vi "MainTagBrowser.vi"() -> ()   [LabVIEW 2020]
doc: "Read Binary File opens and reads an existing file stored as a double precision array in binary form. This VI shows the simplest way to read this entire file, with the simplest error checking."
panel:
  in  "Tag List":i32(listbox)=-1
  out "TagValue":string
  out "TagName":string
  out "TagType":string
  in  "Tag_num":i32 min=0 max=106
  out "n_hdr_items":i32=80
  out "file error status":errorcluster
  out "Version":string
  out "Magic":string
  # "Select the tag number here and see the content below"
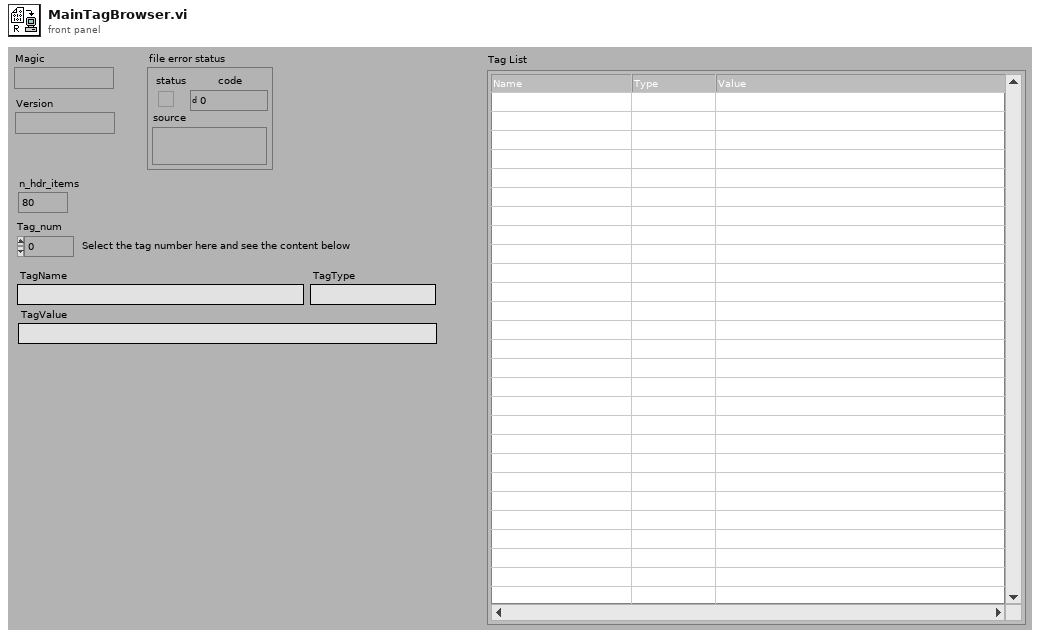
[diagram p1: front panel]
types:
  T1 = cluster{"TagIdent":string, "TagIndex":i32, "TagType":i32, "TagValue":i64, "TagAuxData":string}
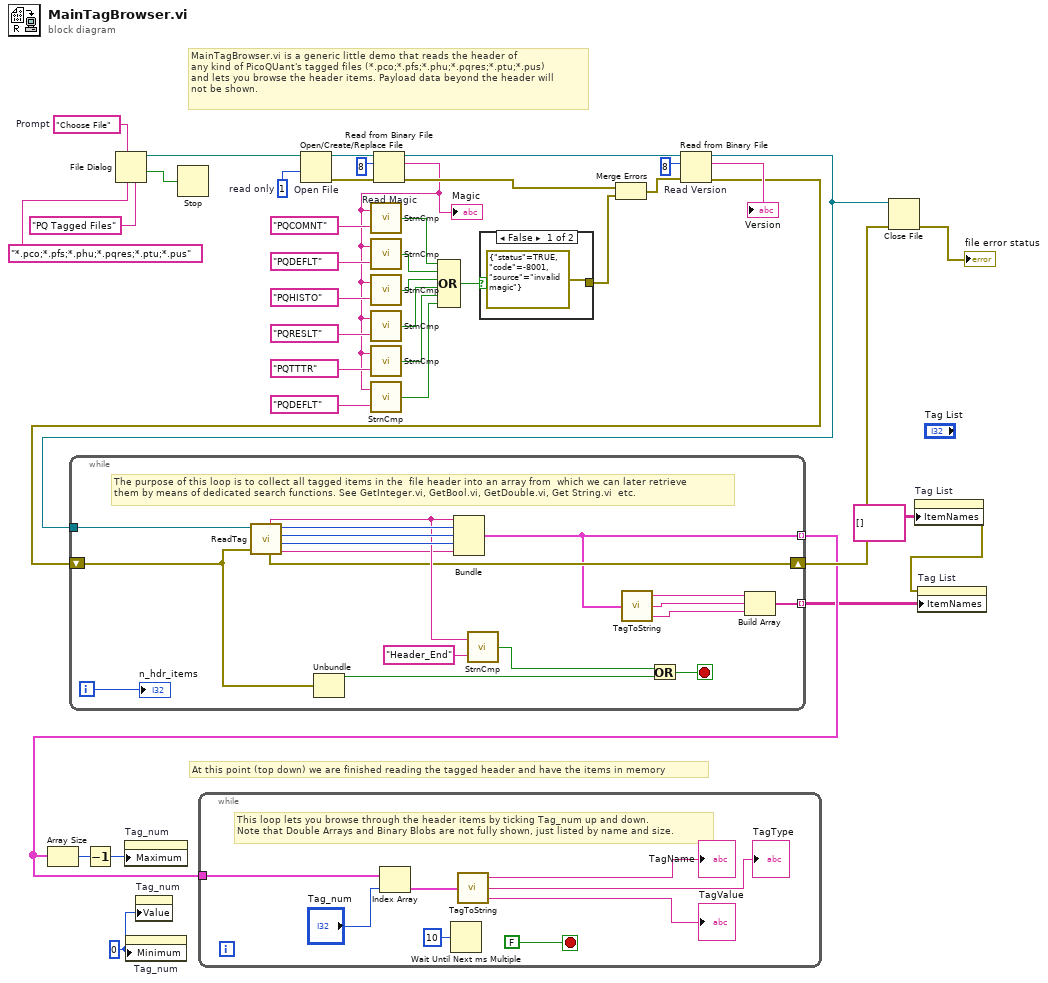
[diagram p0: block diagram]
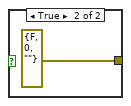
[diagram p2: hidden frame]
diagram:
  w5 = 0
  w4 = 1  # read only
  w39 = "Choose File"  # Prompt
  # "MainTagBrowser.vi is a generic little demo that reads the header of\nany kind of PicoQUant's tagged files (*.pco;*.pfs;*.phu;*.pqres;*.ptu;*.pus)\nand lets you browse the header items. Payload data beyond the header will \nnot be shown."
  # "At this point (top down) we are finished reading the tagged header and have the items in memory"
  n1 = File Dialog(4:"PQ Tagged Files", 6:"*.pco;*.pfs;*.phu;*.pqres;*.ptu;*.pus", 7:w39) -> (1:w27:bool, 3:w40:path)  [unwired: 4 in, 2 out]
  n2 = property on="Tag_num" class="DigNum (strict)"("Minimum"=w5) -> ()  [unwired: 2 in, 2 out]
  n3 = property on="Tag_num" class="DigNum (strict)"("Value"=w5) -> ()  [unwired: 2 in, 2 out]
  n4 = Stop(stop? (T)=w27) -> ()
  n5 = Open/Create/Replace File "Open File"(file path (use dialog)=w40, access (0:read/write)=w4) -> (refnum out=w29:refnum<file>, error out=w28:errorcluster)  [unwired: 4 in, 1 out]
  n6 = Read from Binary File "Read Magic"(8:w28, 10:8, 11:w29) -> (0:w33:errorcluster, 2:w9:string, 3:w38:refnum<file>)  [unwired: 3 in, 1 out]
  "Magic" <- w9
  n7 = call "StrnCmp.vi"("String 2"="PQCOMNT", "String 1"=w9) -> ("equal"=w16:bool)
  n8 = call "StrnCmp.vi"("String 2"="PQDEFLT", "String 1"=w9) -> ("equal"=w15:bool)
  n9 = call "StrnCmp.vi"("String 2"="PQHISTO", "String 1"=w9) -> ("equal"=w14:bool)
  n10 = call "StrnCmp.vi"("String 2"="PQRESLT", "String 1"=w9) -> ("equal"=w13:bool)
  n11 = call "StrnCmp.vi"("String 2"="PQTTTR", "String 1"=w9) -> ("equal"=w12:bool)
  n12 = call "StrnCmp.vi"("String 2"="PQDEFLT", "String 1"=w9) -> ("equal"=w11:bool)
  n13 = Compound Arithmetic op=OR(w16, w15, w14, w13, w12, w11) -> (w10:bool)
  n14 = case shown="False" w10 {
    tunnel: [errorcluster {"status"=TRUE, "code"=-8001, "source"="invalid magic"} ("file error status 2") errorcluster {"status"=FALSE, "code"=0, "source"=""} ("file error status 2")] -> w31
    frame False {
    }
    frame True {
    }
  }
  n15 = Merge Errors(w33, w31) -> (w32:errorcluster)
  n16 = Read from Binary File "Read Version"(8:w32, 10:8, 11:w38) -> (0:w26:errorcluster, 2:→"Version":string, 3:w24:refnum<file>)  [unwired: 3 in, 1 out]
  n17 = while {
    shift-left: w26 -> [w58]
    shift-right: [w48] -> w25
    tunnel: w24 -> [w60]
    tunnel: [w47] -> w8 mode=indexing
    tunnel: [w43] -> w3 mode=indexing
    i -> [w54]
    stop <- w59 stop-if-true
    # "The purpose of this loop is to collect all tagged items in the  file header into an array from  which we can later retrieve \nthem by means of dedicated search functions. See GetInteger.vi, GetBool.vi, GetDouble.vi, Get String.vi  etc."
    n18 = call "ReadTag.vi"("refnum"=w60, "error in"=w58) -> ("TagIdent"=w50:string, "TagIndex"=w57:i32, "TagType"=w56:i32, "error out"=w48:errorcluster, "TagValue"=w55:i64, "TagAuxData"=w49:string)  [unwired: 3 in]
    n19 = Unbundle(w58) -> ("status"=w51:bool)  [unwired: 2 out]
    n20 = Bundle("TagIdent"=w50, "TagIndex"=w57, "TagType"=w56, "TagValue"=w55, "TagAuxData"=w49) -> (w47:T1)  [unwired: 1 in]
    n21 = call "StrnCmp.vi"("String 2"="Header_End", "String 1"=w50) -> ("equal"=w52:bool)
    n22 = call "TagToString.vi"("TagData"=w47) -> ("StrTagValue"=w44:string, "StrTagType"=w45:string, "StrTagName"=w46:string)  [unwired: 2 in]
    n23 = Or(x=w52, y=w51) -> (x .or. y?=w59:bool)
    n24 = Build Array(w46, w45, w44) -> (w43:string[])
    "n_hdr_items" <- w54
  }
  n25 = Array Size(array=w8) -> (size(s)=w7:i32)
  n26 = Decrement(x=w7) -> (x-1=w6:i32)
  n27 = property on="Tag_num" class="DigNum (strict)"("Maximum"=w6) -> ()  [unwired: 2 in, 2 out]
  n28 = while {
    tunnel: w8 -> [w67]
    stop <- FALSE stop-if-true
    # "This loop lets you browse through the header items by ticking Tag_num up and down.\nNote that Double Arrays and Binary Blobs are not fully shown, just listed by name and size."
    n29 = Index Array(array=w67, index="Tag_num") -> (element=w65:T1)
    n30 = Wait Until Next ms Multiple(millisecond multiple=u32 10) -> ()  [unwired: 1 out]
    n31 = call "TagToString.vi"("TagData"=w65) -> ("StrTagValue"=→"TagValue":string, "StrTagType"=→"TagType":string, "StrTagName"=→"TagName":string)  [unwired: 2 in]
  }
  n32 = Close File(refnum=w24, error in=w25) -> (error out=→"file error status":errorcluster)  [unwired: 1 out]
  n33 = property on="Tag List" class="MCListbox (strict)"("ItemNames"=string[][] [] ("Item Names")) -> (error out=w2:errorcluster)  [unwired: 2 in, 1 out]
  n34 = property on="Tag List" class="MCListbox (strict)"(error in=w2, "ItemNames"=w3) -> ()  [unwired: 1 in, 2 out]
